vi "getThreshConv.vi"(7 "format string":string, 10 "error in (no error)":errorcluster, 11 "Input HEX Threshold":string) -> (2 "error out":errorcluster, 3 "Output Threshold Value":u16, 5 "Raw Data":u16)   [LabVIEW 2019]
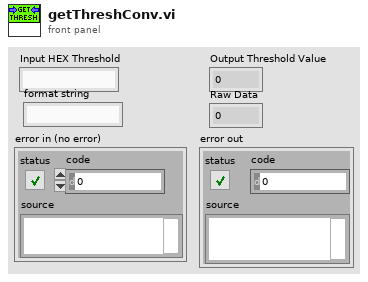
[diagram p1: front panel]
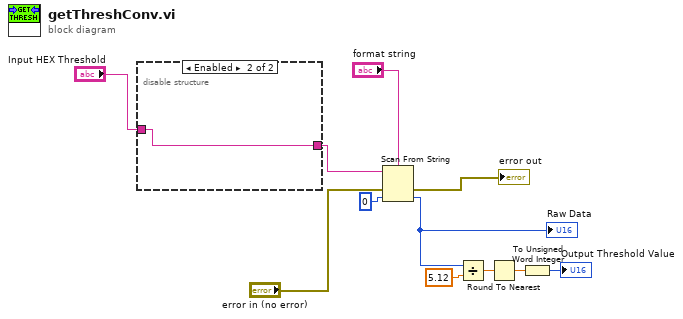
[diagram p0: block diagram]
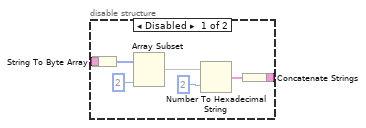
[diagram p2: hidden frame]
diagram:
  n1 = disable-structure shown="Enabled" {
    disable-tunnel: "Input HEX Threshold" -> [w18 w19]
    disable-tunnel: [w17 w19] -> w4
    frame Disabled {
      n2 = String To Byte Array(string=w18) -> (unsigned byte array=w14:u8[])
      n3 = Array Subset(array=w14, length=2) -> (w13:u8[])  [unwired: 1 in]
      n4 = Number To Hexadecimal String(1:i16 2 ("Breite (-)"), 2:w13) -> (0:w16:string[])
      n5 = Concatenate Strings(w16) -> (w17:string)
    }
    frame Enabled {
    }
  }
  n6 = Scan From String(format string="format string", input string=w4, error in="error in (no error)", default 1=u16 0 ("default value 1")) -> (error out=→"error out":errorcluster, output 1=w6:u16)  [unwired: 1 in, 2 out]
  "Raw Data" <- w6
  n7 = Divide(x=w6, y=5.12) -> (x/y=w9:dbl)
  n8 = Round To Nearest(number=w9) -> (nearest integer value=w3:dbl)
  n9 = To Unsigned Word Integer(number=w3) -> (unsigned 16bit integer=→"Output Threshold Value":u16)
